vi "cv.to.local_publisher.vi"(8 "error in (no error)":errorcluster, 11 "cv publisher":T1) -> (0 "error out":errorcluster, 3 "local publisher":T4)   [LabVIEW 2024, in "CV_RESTful_Lib.lvlib"]
uses:
  CV_RESTful_Lib.lvlib
  typedefs/local_publisher--cluster.ctl
  typedefs/cv_publisher--cluster.ctl
  typedefs/cv_publisher.results--cluster.ctl
  typedefs/cv_volume.issue--cluster.ctl
  <userlib>/_OpenG.lib/string/string.llb/openg_string.lvlib
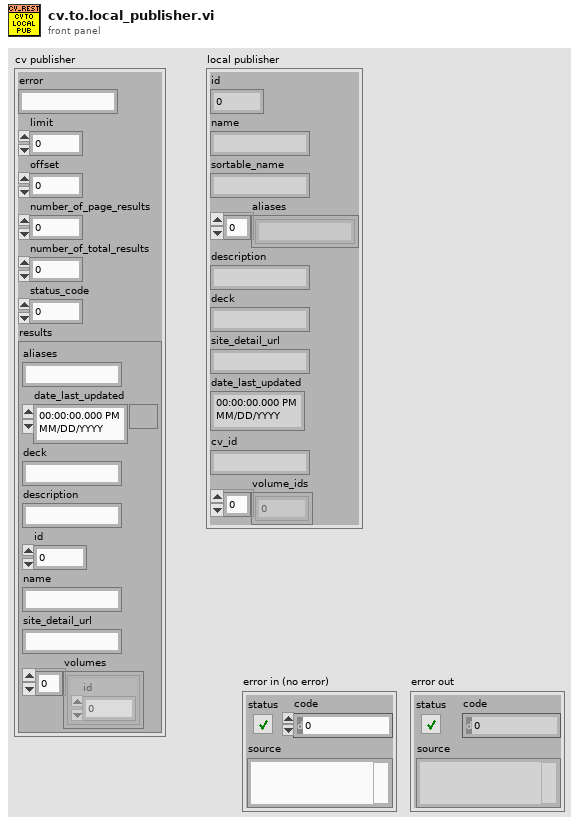
[diagram p1: front panel]
types:
  T1 = typedef "CV_RESTful_Lib.lvlib/cv_publisher--cluster.ctl" = cluster{"error":string, "limit":i32, "offset":i32, "number_of_page_results":i32, "number_of_total_results":i32, "status_code":i32, "results":T2}
  T2 = typedef "CV_RESTful_Lib.lvlib/cv_publisher.results--cluster.ctl" = cluster{"aliases":string, "date_last_updated":timestamp, "deck":string, "description":string, "id":i32, "name":string, "site_detail_url":string, "volumes":T3[]}
  T3 = typedef "CV_RESTful_Lib.lvlib/cv_volume.issue--cluster.ctl" = cluster{"id":i32}
  T4 = typedef "CV_RESTful_Lib.lvlib/local_publisher--cluster.ctl" = cluster{"id":i32, "name":string, "sortable_name":string, "aliases":string[], "description":string, "deck":string, "site_detail_url":string, "date_last_updated":timestamp, "cv_id":string, "volume_ids":i32[]}
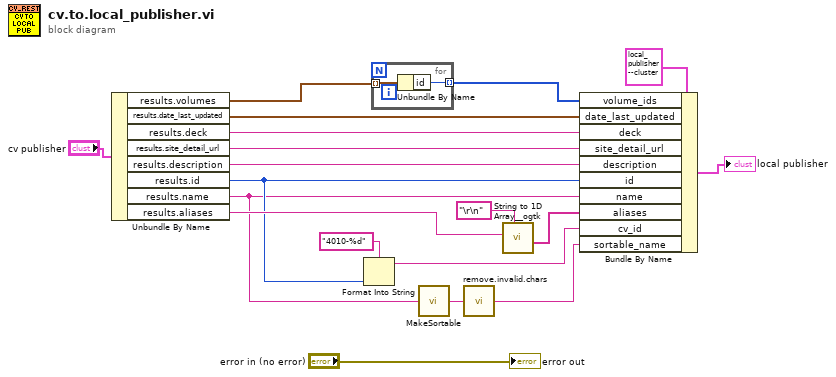
[diagram p0: block diagram]
diagram:
  n1 = Unbundle By Name("cv publisher") -> ("results.volumes"=w2:T3[], "results.date_last_updated"=w3:timestamp, "results.deck"=w5:string, "results.site_detail_url"=w11:string, "results.description"=w12:string, "results.id"=w9:i32, "results.name"=w6:string, "results.aliases"=w15:string)
  n2 = Format Into String(format string="4010-%d", w9) -> (resulting string=w8:string)  [unwired: 2 in, 1 out]
  n3 = for {
    tunnel: w2 -> [w21] mode=indexing
    tunnel: [w20] -> w1 mode=indexing
    n4 = Unbundle By Name(w21) -> ("id"=w20:i32)
  }
  n5 = call "MakeSortable.vi"("string in"=w6) -> ("string out"=w16:string)
  n6 = call "remove.invalid.chars.vi"("string in"=w16) -> ("string out"=w4:string)
  n7 = call <userlib>:"String to 1D Array__ogtk.vi"("delimiter (Tab)"="\r\n", "string"=w15) -> ("Array of Strings"=w13:string[])  [unwired: 9 in]
  n8 = Bundle By Name(cluster=T4 {"id"=0, "name"="", "sortable_name"="", "aliases"=[], "description"="", "deck"="", "site_detail_url"="", "date_last_updated"=timestamp(0 s since 1904-01-01), "cv_id"="", "volume_ids"=[]} ("local publisher"), "volume_ids"=w1, "date_last_updated"=w3, "deck"=w5, "site_detail_url"=w11, "description"=w12, "id"=w9, "name"=w6, "aliases"=w13, "cv_id"=w8, "sortable_name"=w4) -> (→"local publisher":T4)
  "error out" <- "error in (no error)"
